vi "Comparación de colores.vi"(0 "Color Spectrum":dbl[](array[numeric]) format="%.2f", 1 "Color Spectrum 2":dbl[](array[numeric]) format="%.2f", 2 "Color Spectrum 3":dbl[](array[numeric]) format="%.2f", 3 "Color Spectrum 4":dbl[](array[numeric]) format="%.2f", 4 "Color Spectrum 5":dbl[](array[numeric]) format="%.2f", 5 "Color Spectrum 6":dbl[](array[numeric]) format="%.2f", 6 "Color Spectrum 7":dbl[](array[numeric]) format="%.2f", 7 "Color Spectrum 8":dbl[](array[numeric]) format="%.2f") -> ()   [LabVIEW 2021]
panel:
  in  "Bandera Persona 8":bool
  in  "Bandera Obstaculo 8":bool
  in  "Bandera Obstaculo 7":bool
  in  "Bandera Obstaculo 6":bool
  in  "Bandera Obstaculo 5":bool
  in  "Bandera Obstaculo 4":bool
  in  "Bandera Obstaculo 3":bool
  in  "Bandera Obstaculo 2":bool
  in  "Bandera Obstaculo 1":bool
  in  "Bandera Persona 7":bool
  in  "Bandera Persona 6":bool
  in  "Bandera Persona 5":bool
  in  "Bandera Persona 4":bool
  in  "Bandera Persona 3":bool
  in  "Bandera Persona 2":bool
  in  "Bandera Persona 1":bool
  in  "lower limit":dbl
  in  "upper limit":dbl
  in  "ROI Rojo":i32
  in  "ROI Azul":i32
  # "Elementos de depuración"
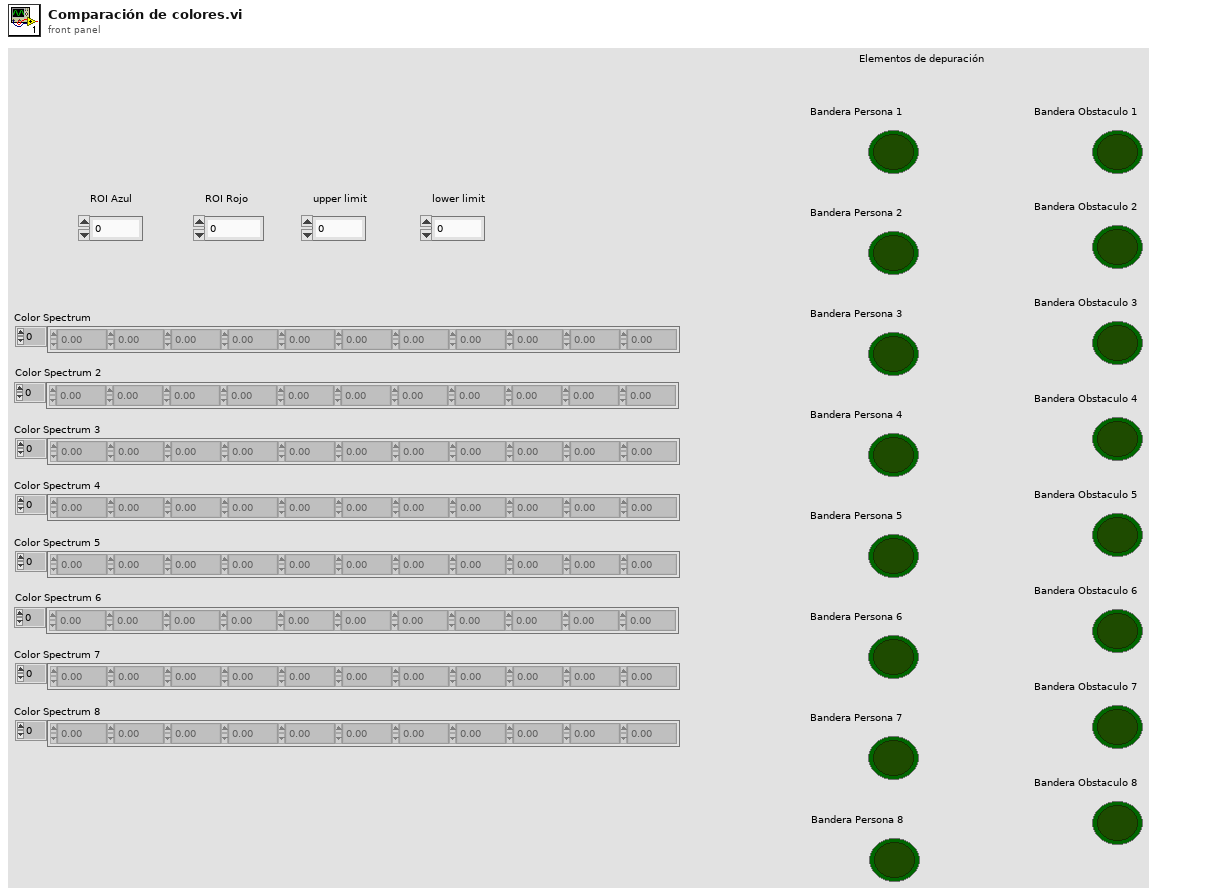
[diagram p1: front panel]
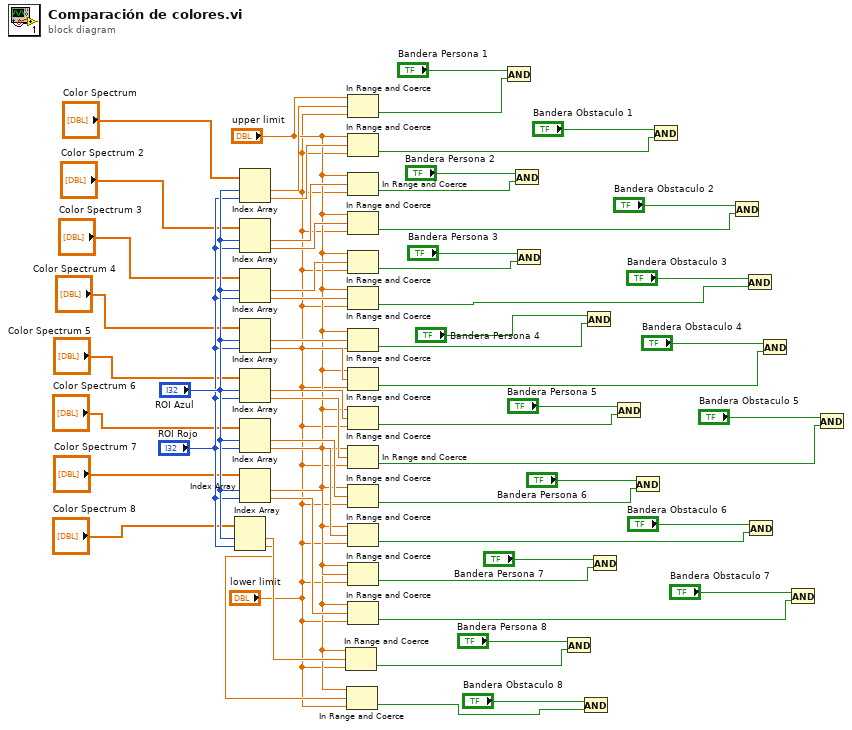
[diagram p0: block diagram]
diagram:
  n1 = Index Array(array="Color Spectrum 8", index #1="ROI Azul", index #2="ROI Rojo") -> (element #1=w43:dbl, element #2=w42:dbl)
  n2 = Index Array(array="Color Spectrum", index #1="ROI Azul", index #2="ROI Rojo") -> (element #1=w55:dbl, element #2=w54:dbl)
  n3 = Index Array(array="Color Spectrum 2", index #1="ROI Azul", index #2="ROI Rojo") -> (element #1=w53:dbl, element #2=w52:dbl)
  n4 = Index Array(array="Color Spectrum 3", index #1="ROI Azul", index #2="ROI Rojo") -> (element #1=w51:dbl, element #2=w50:dbl)
  n5 = Index Array(array="Color Spectrum 4", index #1="ROI Azul", index #2="ROI Rojo") -> (element #1=w49:dbl, element #2=w48:dbl)
  n6 = Index Array(array="Color Spectrum 5", index #1="ROI Azul", index #2="ROI Rojo") -> (element #1=w47:dbl, element #2=w46:dbl)
  n7 = Index Array(array="Color Spectrum 6", index #1="ROI Azul", index #2="ROI Rojo") -> (element #1=w45:dbl, element #2=w44:dbl)
  n8 = Index Array(array="Color Spectrum 7", index #1="ROI Azul", index #2="ROI Rojo") -> (element #1=w60:dbl, element #2=w56:dbl)
  n9 = In Range and Coerce(upper limit="upper limit", x=w43, lower limit="lower limit") -> (In Range?=w17:bool)  [unwired: 1 out]
  n10 = In Range and Coerce(upper limit="upper limit", x=w42, lower limit="lower limit") -> (In Range?=w1:bool)  [unwired: 1 out]
  n11 = In Range and Coerce(upper limit="upper limit", x=w55, lower limit="lower limit") -> (In Range?=w32:bool)  [unwired: 1 out]
  n12 = In Range and Coerce(upper limit="upper limit", x=w54, lower limit="lower limit") -> (In Range?=w8:bool)  [unwired: 1 out]
  n13 = In Range and Coerce(upper limit="upper limit", x=w53, lower limit="lower limit") -> (In Range?=w30:bool)  [unwired: 1 out]
  n14 = In Range and Coerce(upper limit="upper limit", x=w52, lower limit="lower limit") -> (In Range?=w7:bool)  [unwired: 1 out]
  n15 = In Range and Coerce(upper limit="upper limit", x=w51, lower limit="lower limit") -> (In Range?=w28:bool)  [unwired: 1 out]
  n16 = In Range and Coerce(upper limit="upper limit", x=w50, lower limit="lower limit") -> (In Range?=w6:bool)  [unwired: 1 out]
  n17 = In Range and Coerce(upper limit="upper limit", x=w49, lower limit="lower limit") -> (In Range?=w22:bool)  [unwired: 1 out]
  n18 = In Range and Coerce(upper limit="upper limit", x=w48, lower limit="lower limit") -> (In Range?=w5:bool)  [unwired: 1 out]
  n19 = In Range and Coerce(upper limit="upper limit", x=w47, lower limit="lower limit") -> (In Range?=w21:bool)  [unwired: 1 out]
  n20 = In Range and Coerce(upper limit="upper limit", x=w46, lower limit="lower limit") -> (In Range?=w4:bool)  [unwired: 1 out]
  n21 = In Range and Coerce(upper limit="upper limit", x=w45, lower limit="lower limit") -> (In Range?=w20:bool)  [unwired: 1 out]
  n22 = In Range and Coerce(upper limit="upper limit", x=w44, lower limit="lower limit") -> (In Range?=w3:bool)  [unwired: 1 out]
  n23 = In Range and Coerce(upper limit="upper limit", x=w60, lower limit="lower limit") -> (In Range?=w19:bool)  [unwired: 1 out]
  n24 = In Range and Coerce(upper limit="upper limit", x=w56, lower limit="lower limit") -> (In Range?=w2:bool)  [unwired: 1 out]
  n25 = And(x="Bandera Persona 1", y=w32) -> ()  [unwired: 1 out]
  n26 = And(x="Bandera Persona 2", y=w30) -> ()  [unwired: 1 out]
  n27 = And(x="Bandera Persona 3", y=w28) -> ()  [unwired: 1 out]
  n28 = And(x="Bandera Persona 8", y=w17) -> ()  [unwired: 1 out]
  n29 = And(x="Bandera Obstaculo 8", y=w1) -> ()  [unwired: 1 out]
  n30 = And(x="Bandera Persona 4", y=w22) -> ()  [unwired: 1 out]
  n31 = And(x="Bandera Persona 7", y=w19) -> ()  [unwired: 1 out]
  n32 = And(x="Bandera Persona 5", y=w21) -> ()  [unwired: 1 out]
  n33 = And(x="Bandera Persona 6", y=w20) -> ()  [unwired: 1 out]
  n34 = And(x="Bandera Obstaculo 1", y=w8) -> ()  [unwired: 1 out]
  n35 = And(x="Bandera Obstaculo 2", y=w7) -> ()  [unwired: 1 out]
  n36 = And(x="Bandera Obstaculo 3", y=w6) -> ()  [unwired: 1 out]
  n37 = And(x="Bandera Obstaculo 6", y=w3) -> ()  [unwired: 1 out]
  n38 = And(x="Bandera Obstaculo 4", y=w5) -> ()  [unwired: 1 out]
  n39 = And(x="Bandera Obstaculo 7", y=w2) -> ()  [unwired: 1 out]
  n40 = And(x="Bandera Obstaculo 5", y=w4) -> ()  [unwired: 1 out]
